vi "DQMH_close modules.vi"(11 "Modules":T1) -> ()   [LabVIEW 2025]
uses:
  Libraries/USB IO/USB IO.lvlib
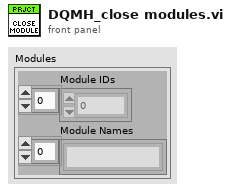
[diagram p1: front panel]
types:
  T1 = cluster{"Module IDs":i32[], "Module Names":string[]}
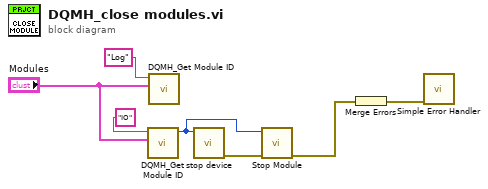
[diagram p0: block diagram]
diagram:
  n1 = call "DQMH_Get Module ID.vi"("Modules"="Modules", "Module Name"="IO") -> ("Module ID out"=w1:i32)  [unwired: 9 in]
  n2 = call "DQMH_Get Module ID.vi"("Modules"="Modules", "Module Name"="Log") -> ()  [unwired: 9 in, 1 out]
  n3 = call "stop device.vi"("Module ID"=w1) -> ("error out"=w2:errorcluster)  [unwired: 9 in, 1 out]
  n4 = call "Stop Module.vi"("error in"=w2, "Module ID"=w1) -> ("error out"=w3:errorcluster)  [unwired: 9 in]
  n5 = Merge Errors(w3) -> (w6:errorcluster)
  n6 = call <vilib>:"Simple Error Handler.vi"("error in (no error)"=w6) -> ()  [unwired: 4 in, 5 out]
